vi "转换-时间字符串至数值时间数组.vi"(11 "时分秒(xx:xx:xx)":string) -> (0 "时分秒数组":i32[](array[numeric]), 1 "秒":i32, 2 "分":i32, 3 "时":i32)   [LabVIEW 2013]
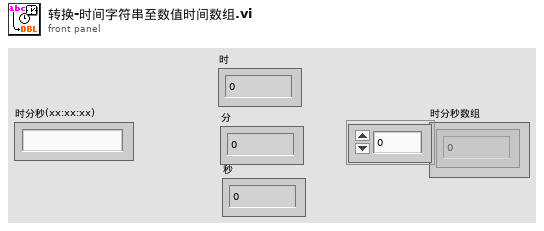
[diagram p1: front panel]
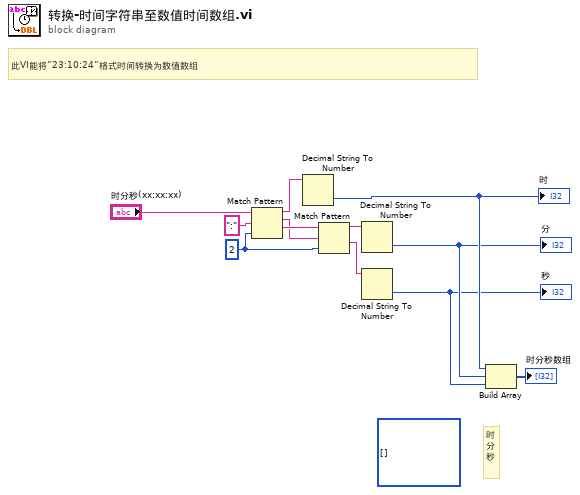
[diagram p0: block diagram]
diagram:
  (unwired) i32[] [] ("添加的数组")
  w1 = 2 ("偏移量(0)")
  # "时\n分\n秒"
  # "此VI能将”23:10:24“格式时间转换为数值数组"
  n1 = Match Pattern(string="时分秒(xx:xx:xx)", regular expression=":" ("正则表达式"), offset (0)=w1) -> (before substring=w8:string, match substring=w9:string, after substring=w10:string)  [unwired: 1 out]
  n2 = Decimal String To Number(string=w8) -> (number=w5:i32)  [unwired: 2 in, 1 out]
  "时" <- w5
  n3 = Match Pattern(string=w10, regular expression=w9, offset (0)=w1) -> (before substring=w7:string, after substring=w6:string)  [unwired: 2 out]
  n4 = Decimal String To Number(string=w7) -> (number=w4:i32)  [unwired: 2 in, 1 out]
  "分" <- w4
  n5 = Decimal String To Number(string=w6) -> (number=w3:i32)  [unwired: 2 in, 1 out]
  "秒" <- w3
  n6 = Build Array(w5, w4, w3) -> (→"时分秒数组":i32[])
